vi "receive.vi"(0 "object in":refnum<class "serial_work.lvclass">, 5 "error in (no error)":errorcluster) -> (14 "object out":refnum<class "serial_work.lvclass">, 15 "读取缓冲区":string, 16 "返回数":u32, 19 "error out":errorcluster)   [LabVIEW 2016, in "serial_work.lvclass"]
uses:
  serial_work.lvclass
  serial_work.lvclass/serial_work.ctl
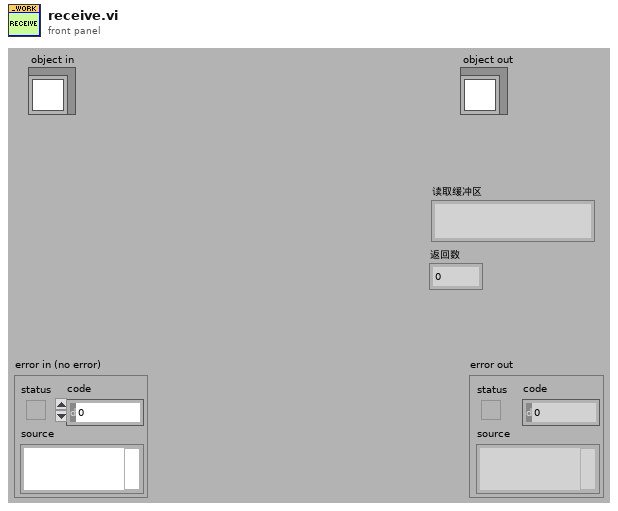
[diagram p1: front panel]
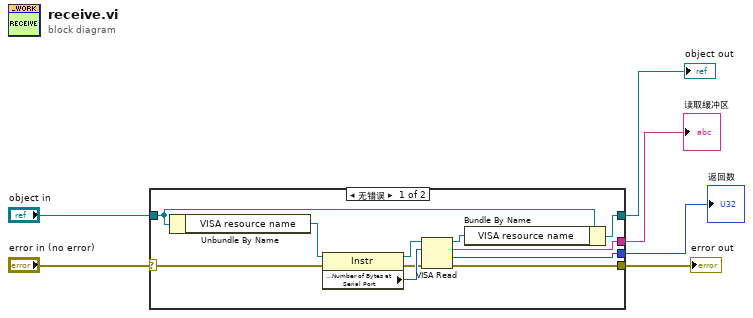
[diagram p0: block diagram]
diagram:
  n1 = case shown="无错误" "error in (no error)" {
    selector: "error in (no error)" -> [w10 w19]
    tunnel: [w9 w19] -> w5
    tunnel: [w16 w18] -> w3
    tunnel: "object in" -> [w17 w18]
    tunnel: [w8 _] -> w2
    tunnel: [w7 _] -> w1
    frame No Error {
      n2 = Unbundle By Name(w17) -> ("VISA resource name"=w12:refnum<visa-resource-name>)
      n3 = property class="Instr"(reference=w12, error in=w10) -> (reference out=w13:refnum<visa-resource-name>, error out=w14:errorcluster, "Serial Settings:Number of Bytes at Serial Port"=w15:u32)
      n4 = VISA Read(VISA resource name=w13, byte count=w15, error in (no error)=w14) -> (VISA resource name out=w11:refnum<visa-resource-name>, read buffer=w8:string, return count=w7:u32, error out=w9:errorcluster)
      n5 = Bundle By Name(cluster=w17, "VISA resource name"=w11) -> (w16:refnum<class "serial_work.lvclass">)
    }
    frame Error {
    }
  }
  "error out" <- w5
  "object out" <- w3
  "读取缓冲区" <- w2
  "返回数" <- w1
